vi "Reset All Grid Tiles.vi"(8 "error in (no error)":errorcluster, 11 "Controller in":refnum<class "Controller.lvclass">) -> (0 "error out":errorcluster, 3 "Controller out":refnum<class "Controller.lvclass">)   [LabVIEW 2021, in "Controller.lvlib" / "Controller.lvclass"]
uses:
  Controller.lvclass
  Controller.lvclass/Controller.ctl
  MC Screen/Grid Screen Messages/Reset Board Appearance Msg/Reset Board Appearance Msg.lvclass/Reset Board Appearance Msg.ctl
  <vilib>/ActorFramework/Message Enqueuer/Message Enqueuer.lvclass/Message Enqueuer.ctl
  <vilib>/ActorFramework/Message Enqueuer/Enqueue.vi
  MC Screen/Grid Screen Messages/Reset Board Appearance Msg/Reset Board Appearance Msg.lvclass
  C:/Program Files/National Instruments/LabVIEW 2024/vi.lib/ActorFramework/Message/Message.lvclass
  <vilib>/ActorFramework/Message Priority Queue/Priority Enqueue.vi
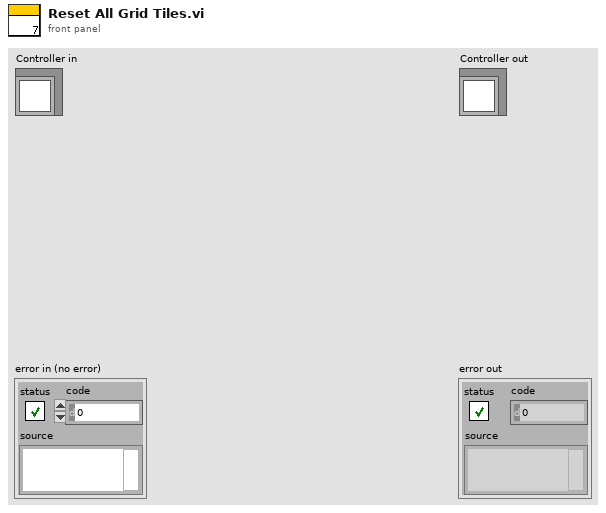
[diagram p1: front panel]
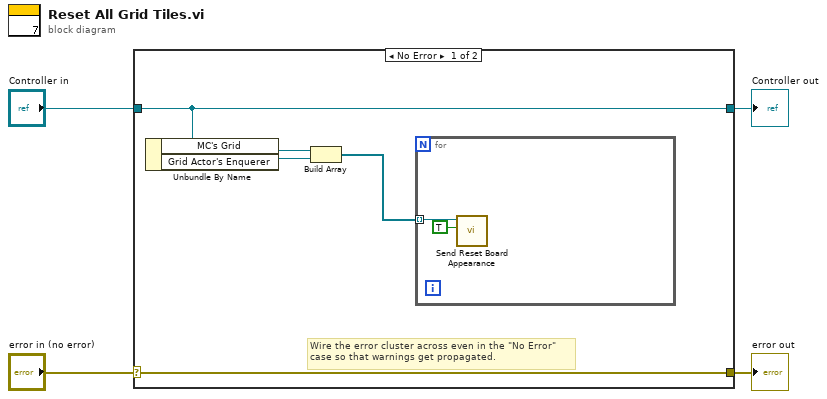
[diagram p0: block diagram]
diagram:
  n1 = case shown="No Error" "error in (no error)" {
    selector: "error in (no error)" -> [w9 w13]
    tunnel: [w9 w13] -> w3
    tunnel: [w8 w12] -> w1
    tunnel: "Controller in" -> [w8 w12]
    frame No Error {
      # "Wire the error cluster across even in the \"No Error\"\ncase so that warnings get propagated."
      n2 = Unbundle By Name(w8) -> ("MC's Grid"=w6:refnum<class "Message Enqueuer.lvclass">, "Grid Actor's Enquerer"=w7:refnum<class "Message Enqueuer.lvclass">)
      n3 = Build Array(w6, w7) -> (w5:refnum<class "Message Enqueuer.lvclass">[])
      n4 = for {
        tunnel: w5 -> [w11] mode=indexing
        n5 = call "Send Reset Board Appearance.vi"("Value"=TRUE, "Message Enqueuer"=w11) -> ()  [unwired: 8 in, 2 out]
      }
    }
    frame Error {
    }
  }
  "error out" <- w3
  "Controller out" <- w1
